vi "Configure Pulse.vi"(6 "Delay  (0 s)":dbl format="%#_6f", 8 "error in (no error)":errorcluster, 9 "Width (0.02 s)":dbl=0.02 format="%#_6f", 10 "Period (0.025 s)":dbl=0.025, 11 "VISA resource name":refnum<visa-resource-name>) -> (0 "error out":errorcluster, 3 "VISA resource name out":refnum<visa-resource-name>)   [LabVIEW 2015, in "Fluke 28x Series.lvlib"]
doc: "Configures a single pulse signal. This is one of the standard waveforms that can be output by the generator."
uses:
  <instrlib>/Fluke 28x Series/Fluke 28x Series.lvlib
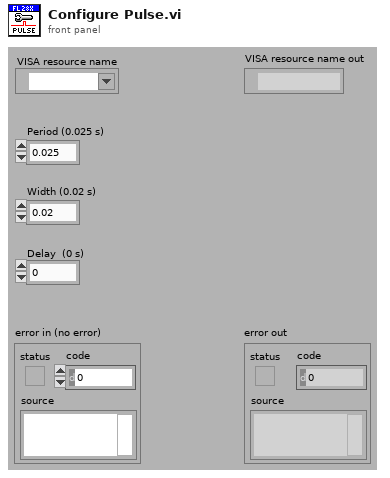
[diagram p1: front panel]
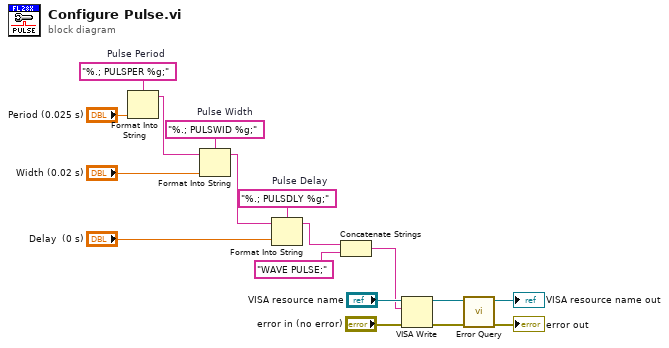
[diagram p0: block diagram]
diagram:
  w12 = "%.; PULSDLY %g;"  # Pulse Delay
  w15 = "%.; PULSWID %g;"  # Pulse Width
  w17 = "%.; PULSPER %g;"  # Pulse Period
  n1 = Format Into String(format string=w17, "Period (0.025 s)") -> (resulting string=w13:string)  [unwired: 2 in, 1 out]
  n2 = Format Into String(format string=w15, initial string=w13, "Width (0.02 s)") -> (resulting string=w11:string)  [unwired: 1 in, 1 out]
  n3 = Format Into String(format string=w12, initial string=w11, "Delay  (0 s)") -> (resulting string=w5:string)  [unwired: 1 in, 1 out]
  n4 = Concatenate Strings(w5, "WAVE PULSE;" ("string")) -> (w3:string)
  n5 = VISA Write(VISA resource name="VISA resource name", write buffer=w3, error in (no error)="error in (no error)") -> (VISA resource name out=w8:refnum<visa-resource-name>, error out=w7:errorcluster)  [unwired: 1 out]
  n6 = call <instrlib>:"Error Query.vi"("error in (no error)"=w7, "VISA resource name"=w8) -> ("error out"=→"error out":errorcluster, "VISA resource name out"=→"VISA resource name out":refnum<visa-resource-name>)  [unwired: 6 in, 2 out]
